vi "DN4_Counter_SetFrequency_Ex.vi"(3 "error in (no error)":errorcluster, 4 "frequency":dbl[](array[numeric]), 5 "Task ID":u32) -> (0 "error out":errorcluster, 2 "Task ID":u32)   [LabVIEW 2009]
uses:
  Windows/System32/AdvLvDaq.dll
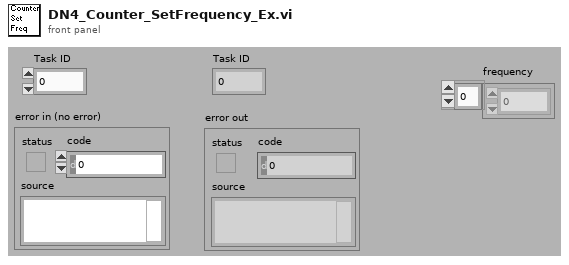
[diagram p1: front panel]
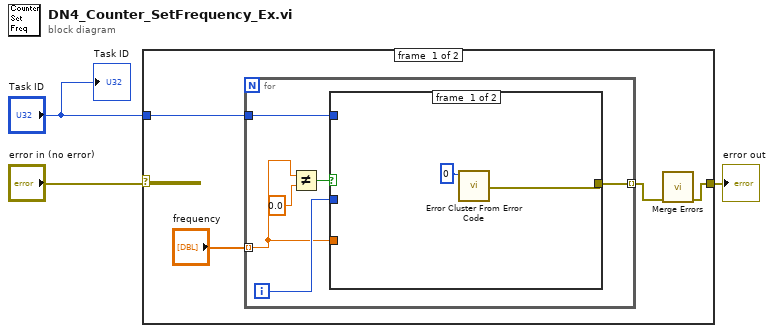
[diagram p0: block diagram]
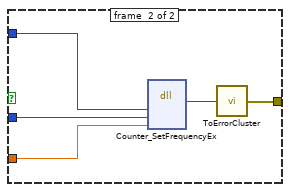
[diagram p2: hidden frame]
diagram:
  n1 = case shown="No Error" "error in (no error)" {
    selector: "error in (no error)" -> [_ w21]
    tunnel: "Task ID" -> [w6 _]
    tunnel: [w5 w21] -> w2
    frame #0 {
      n2 = for {
        tunnel: [w11] -> w4 mode=indexing
        tunnel: "frequency" -> [w8] mode=indexing
        tunnel: w6 -> [w10]
        i -> [w9]
        n3 = Not Equal?(x=w8, y=0.0) -> (x != y?=w12:bool)
        n4 = case shown="True" w12 {
          tunnel: [w14 w19] -> w11
          tunnel: w10 -> [_ w18]
          tunnel: w9 -> [_ w17]
          tunnel: w8 -> [_ w16]
          frame #0 {
            n5 = call <vilib>:"Error Cluster From Error Code.vi"("error code (0)"=0) -> ("error out"=w14:errorcluster)  [unwired: 2 in, 6 out]
          }
          frame #1 {
            n6 = dll-call lib="C:/Windows/System32/AdvLvDaq.dll" fn="Counter_SetFrequencyEx"("taskId"=w18, "channelIndex"=w17, "frequency"=w16) -> ("return type"=w20:i32)  [unwired: 6 in, 2 out]
            n7 = call <userlib>:"ToErrorCluster.vi"("error code"=w20) -> ("error out"=w19:errorcluster)
          }
        }
      }
      n8 = call <vilib>:"Merge Errors.vi"("error array in"=w4) -> ("error out"=w5:errorcluster)  [unwired: 3 in, 3 out]
    }
    frame #1 {
    }
  }
  "error out" <- w2
  "Task ID" <- "Task ID"
